vi "Read configuration.vi"(8 "error in (no error)":errorcluster, 11 "HiPOT Channel":refnum<class "HiPOT Channel.lvclass">) -> (0 "error out":errorcluster, 2 "configuration":refnum<class "CEF_serializable configuration.lvclass">, 3 "HiPOT Channel out":refnum<class "HiPOT Channel.lvclass">)   [LabVIEW 2025, in "HiPOT.lvlib" / "HiPOT Channel.lvclass"]
uses:
  HiPOT Channel.lvclass
  Users/Public/Documents/Sandia National Labs/TSS Plugin/CEF.lvlibp/serializable configuration/CEF_serializable configuration.lvclass
  HiPOT Channel.lvclass/HiPOT Channel.ctl
  Users/Public/Documents/Sandia National Labs/TSS Plugin/Abstract PlugIn.lvlibp/Plugin/Abstract/Channel configuration/Channel configuration.lvclass
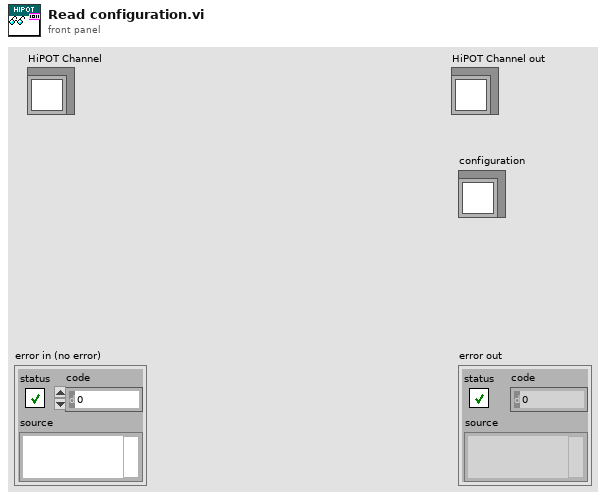
[diagram p1: front panel]
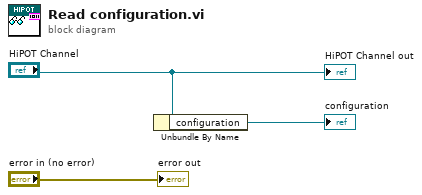
[diagram p0: block diagram]
diagram:
  n1 = Unbundle By Name("HiPOT Channel") -> ("configuration"=→"configuration":refnum<class "Channel configuration.lvclass">)
  "error out" <- "error in (no error)"
  "HiPOT Channel out" <- "HiPOT Channel"
